vi "Tx Inline Start.vi"(8 "error in (no error)":errorcluster, 11 "Framework in":refnum<class "Framework.lvclass">) -> (0 "error out":errorcluster, 3 "Framework out":refnum<class "Framework.lvclass">)   [LabVIEW 2017, in "DSF Core.lvlib" / "Framework.lvclass"]
uses:
  Framework.lvclass
  Framework.lvclass/Framework.ctl
  Plugin/Plugin.lvclass/Plugin.ctl
  Transfer Group/Transfer Group.lvclass/Transfer Group.ctl
  Timing/Timing.lvclass/Timing.ctl
  Buffers/Buffers.lvclass/Buffers.ctl
  <vilib>/NI/Memory Manager/Classes/Pointer/Pointer.lvclass/Pointer.ctl
  Interfaces/Interface/Interface.lvclass/Interface.ctl
  Transfer Group/Increment Iteration.vi
  Transfer Group/Copy Inline to Async.vi
  Transfer Group/Get Iteration.vi
  Dispatcher/Dispatch Transfer Group.vi
  Transfer Group/Get ID.vi
  Plugin/Get ID.vi
  Timing/Increment Iteration.vi
  Buffers/Copy Inline to Async.vi
  Timing/Get Iteration.vi
  Interfaces/Dispatcher/Send Dispatcher Command.vi
  <vilib>/NI/Memory Manager/Classes/Pointer/Copy All.vi
  Interfaces/Dispatcher/Write.vi
  Interfaces/Dispatcher/Write Dispatcher Command.vi
  <vilib>/NI/Memory Manager/Classes/Pointer/Get Size.vi
  <vilib>/NI/Memory Manager/Classes/Pointer/Copy.vi
  Interfaces/Interface/Send Command.vi
  <vilib>/NI/Memory Manager/Classes/Pointer/Copy (No Check).vi
  <vilib>/NI/Memory Manager/Classes/Pointer/Check Pointer Bounds.vi
  <vilib>/NI/Memory Manager/Classes/Pointer/Check Null Pointer.vi
  Interfaces/Interface/Write RT FIFO.vi
  <vilib>/NI/Memory Manager/Classes/Pointer/Get Address.vi
  <vilib>/NI/Memory Manager/Classes/Pointer/Errors.vi
  <vilib>/NI/Memory Manager/Classes/Pointer/Out of Bounds.vi
  <vilib>/NI/Memory Manager/Classes/Pointer/Null Pointer.vi
  <vilib>/NI/Memory Manager/Classes/Pointer/Is Null.vi
  <vilib>/NI/Memory Manager/VIs/Source.Write.String.vi
  <vilib>/NI/Memory Manager/Classes/Pointer/Write Pointer Size.vi
  <vilib>/NI/Memory Manager/Classes/Pointer/Create Error.vi
  <vilib>/NI/Memory Manager/VIs/Source.Write.Scalar.Base10.vi
  <vilib>/NI/Memory Manager/VIs/Source.Write.Scalar.Base10 (U64).vi
  <vilib>/NI/Memory Manager/VIs/New Error Cluster Constant.vi
  <vilib>/NI/Memory Manager/VIs/New Error Cluster Constant (512B).vi
  <vilib>/NI/Memory Manager/VIs/Error Cluster.Set Status.vi
  <vilib>/NI/Memory Manager/VIs/Error Cluster.Set Code.vi
  <vilib>/NI/Memory Manager/VIs/Error Cluster.Set VI Source.vi
  <vilib>/NI/Memory Manager/Constants/Constants.vi
  <vilib>/NI/Memory Manager/Constants/Library Name.vi
  <vilib>/NI/Memory Manager/Classes/Pointer/Pointer Error Info.vi
  <vilib>/NI/Memory Manager/Constants/Pointer Class Name.vi
  Buffer/Buffer.lvclass
  C:/Program Files (x86)/National Instruments/LabVIEW 2017/vi.lib/NI/Memory Manager/Classes/Pointer/Pointer.lvclass
  Interfaces/Dispatcher/Dispatcher Interface.lvclass
  C:/Git/DSF/Data Sharing Framework/Source/Core/Classes/Interfaces/Interface/Interface.lvclass
  Interfaces/Interface/Errors.vi
  Interfaces/Dispatcher/Command Timeout.vi
  VIs/VI Name.vi
  Interfaces/Dispatcher/Class Name.vi
  Plugin/Plugin.lvclass
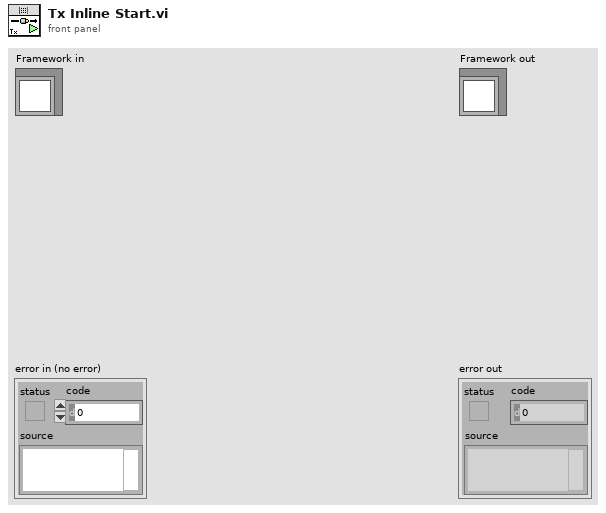
[diagram p1: front panel]
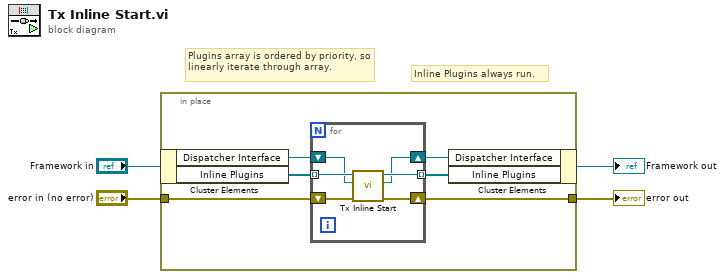
[diagram p0: block diagram]
diagram:
  # "Inline Plugins always run."
  # "Plugins array is ordered by priority, so linearly iterate through array."
  n1 = in-place {
    in-place-border: "error in (no error)" -> [w10]
    in-place-border: [w9] -> w3
    n2 = in-place-cluster #1("Framework in") -> ("Dispatcher Interface"=w6:refnum<class "Dispatcher Interface.lvclass">, "Inline Plugins"=w8:refnum<class "Plugin.lvclass">[])
    n3 = for {
      tunnel: w8 -> [w12] mode=indexing
      tunnel: [w16] -> w7 mode=indexing
      shift-right: [w15] -> w9
      shift-left: w10 -> [w14]
      shift-right: [w13] -> w5
      shift-left: w6 -> [w11]
      n4 = call "Tx Inline Start.vi"("error in (no error)"=w14, "Dispatcher Interface in"=w11, "Plugin in"=w12) -> ("error out"=w15:errorcluster, "Dispatcher Interface out"=w13:refnum<class "Dispatcher Interface.lvclass">, "Plugin out"=w16:refnum<class "Plugin.lvclass">)  [unwired: 6 in]
    }
    n5 = in-place-cluster #1("Dispatcher Interface"=w5, "Inline Plugins"=w7) -> (→"Framework out":refnum<class "Framework.lvclass">)
  }
  "error out" <- w3
